vi "Flatten.vi"(6 "FIFO Timestamps":T1, 8 "error in (no error)":errorcluster, 10 "Data In":refnum<data-value>[](array[refnum]), 11 "CIFTag in":refnum<class "CIF_NIChn_Fifo_DAQ.lvclass">) -> (0 "error out":errorcluster, 2 "Data Out":refnum<data-value>[](array[refnum]), 3 "CIFTag out":refnum<class "CIF_NIChn_Fifo_DAQ.lvclass">)   [LabVIEW 2021, in "CIF_NIChn_Fifo_DAQ.lvclass"]
uses:
  CIF_NIChn_Fifo_DAQ.lvclass
  ChannelCommon/typedef/TimeStamps.ctl
  ChannelCommon/typedef/Datatype Waveform.ctl
  CIF_NIChn_Fifo_DAQ.lvclass/CIF_NIChn_Fifo_DAQ.ctl
  ChannelCommon/CIFFIFO/CIFfifo.lvclass/CIFfifo.ctl
  ChannelCommon/CIFFIFO/Accessors/Write T0.vi
  ChannelCommon/CIFFIFO/Accessors/Write T_Out.vi
  ChannelCommon/CIFFIFO/Accessors/Write ClockID.vi
  <vilib>/CIF Foundation/CIF Utilities/Time/System Time/Get System Time.vi
  ChannelCommon/Utilities/Flatten Header.vi
  <vilib>/CIF Foundation/CIF Utilities/DataTypes/Flatten U64.vi
  ChannelCommon/CIFFIFO/Accessors/Write Payload Length.vi
  ChannelCommon/CIFFIFO/Accessors/Read Header.vi
  <vilib>/CIF Foundation/CIF Utilities/Time/System Time/LabVIEW Time to TAI Time.vi
  <vilib>/CIF Foundation/CIF Utilities/DataTypes/Flatten I64.vi
  D:/dev/Packages/Channel_Manager/src/CIF_NIChn/NIChn/CIF_NIChn.lvclass
  D:/dev/Packages/Channel_Manager/src/CIFChannels/CIFChannels.lvclass
  D:/dev/Packages/Channel_Manager/src/CIF_NIChn/FIFO_DAQ/CIF_NIChn_Fifo_DAQ.lvclass
  ChannelCommon/ChannelCommon.lvlib
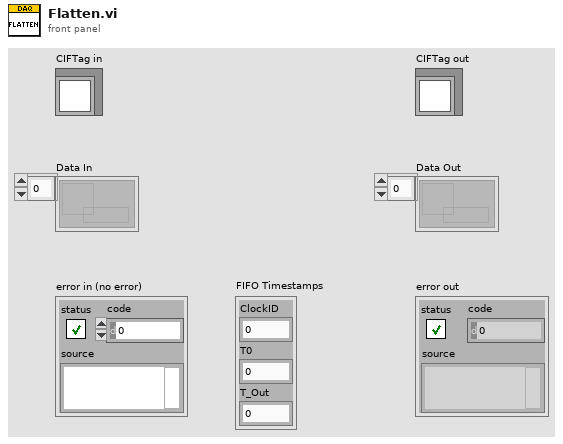
[diagram p1: front panel]
types:
  T1 = typedef "ChannelCommon.lvlib/TimeStamps.ctl" = cluster{"ClockID":u8, "T0":i64, "T_Out":i64}
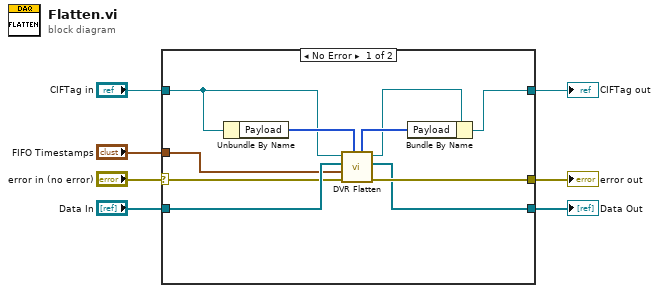
[diagram p0: block diagram]
diagram:
  n1 = case shown="No Error" "error in (no error)" {
    selector: "error in (no error)" -> [w9 w20]
    tunnel: [w17 w20] -> w6
    tunnel: [w16 w19] -> w4
    tunnel: "CIFTag in" -> [w11 w19]
    tunnel: "FIFO Timestamps" -> [w8 _]
    tunnel: "Data In" -> [w15 w18]
    tunnel: [w14 w18] -> w1
    frame No Error {
      n2 = Unbundle By Name(w11) -> ("Payload"=w13:u8[])
      n3 = call "DVR Flatten.vi"("payload in"=w13, "error in (no error)"=w9, "FIFO Timestamps"=w8, "Data In"=w15, "CIFChannels in"=w11) -> ("error out"=w17:errorcluster, "Data Out"=w14:refnum<data-value>[], "CIFChannels out"=w10:refnum<class "CIF_NIChn_Fifo_DAQ.lvclass">, "payload out"=w12:u8[])  [unwired: 2 in, 1 out]
      n4 = Bundle By Name(cluster=w10, "Payload"=w12) -> (w16:refnum<class "CIF_NIChn_Fifo_DAQ.lvclass">)
    }
    frame Error {
    }
  }
  "error out" <- w6
  "CIFTag out" <- w4
  "Data Out" <- w1
